vi "WriteSlowCtrltoH5Test.vi"   [LabVIEW 2012]
uses:
  <vilib>/addons/h5labview2/file/H5Fmode.ctl
  <vilib>/addons/h5labview2/file/H5F.lvlib
  <vilib>/addons/h5labview2/dataset/H5D.lvlib
types:
  T1 = typedef "H5F.lvlib/H5Fmode.ctl" = enum16{"read-only", "read-write", "overwrite", "create new", "open or create"}
  T2 = typedef "hid_t.ctl" = i64
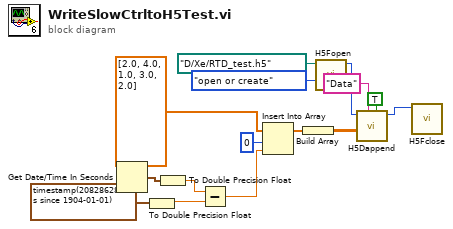
[diagram p0: block diagram]
diagram:
  n1 = Get Date/Time In Seconds() -> (seconds since 1Jan1904=w14:timestamp)
  n2 = To Double Precision Float(number=timestamp(2082862800 s since 1904-01-01)) -> (double precision float=w15:dbl)
  n3 = To Double Precision Float(number=w14) -> (double precision float=w13:dbl)
  n4 = Subtract(x=w13, y=w15) -> (x-y=w12:dbl)
  n5 = Insert Into Array(array=dbl[] [2.0, 4.0, 1.0, 3.0, 2.0] ("Temperatures"), index=0, new element=w12) -> (w9:dbl[])
  n6 = Build Array(w9) -> (w8:dbl[][])
  n7 = call <vilib>:"H5Fopen.vi"("mode (read-only)"=H5Fmode."open or create", "path"=path "D:/Xe/RTD_test.h5") -> ("ref out"=w4:T2)  [unwired: 8 in, 1 out]
  n8 = call <vilib>:"H5Dappend.vi"("create? (T)"=TRUE, "dataset name"="Data", "data"=w8, "ref in"=w4) -> ("ref out"=w3:T2)  [unwired: 4 in, 3 out]
  n9 = call <vilib>:"H5Fclose.vi"("ref"=w3) -> ()  [unwired: 10 in, 1 out]
